vi "DSF.Engine.Builder.Buffer.Parse.vi"(6 "VS Channel Buffer in":dbl[](array[numeric]), 7 "Data Type Buffers in":T5, 8 "error in (no error)":errorcluster, 10 "command":T3, 11 "Builder in":refnum<class "DSF.Engine.Builder.lvclass">) -> (0 "error out":errorcluster, 2 "response":T1, 3 "Builder out":refnum<class "DSF.Engine.Builder.lvclass">, 4 "VS Channel Buffer out":dbl[](array[numeric]), 5 "Data Type Buffers out":T5)   [LabVIEW 2016, in "DSF.Engine.lvlib" / "DSF.Engine.Builder.lvclass"]
uses:
  DSF.Engine.Builder.lvclass
  Typedefs/DSF.Engine.Typedefs.Type Buffers.ctl
  Interface/DSF.Engine.Interface.Builder.Command Data.ctl
  Interface/DSF.Engine.Interface.Builder.Command.ctl
  Interface/DSF.Engine.Interface.Builder.Response Data.ctl
  Interface/DSF.Engine.Interface.Builder.Response.ctl
  DSF.Engine.Builder.lvclass/DSF.Engine.Builder.ctl
  Cache/DSF.Engine.Memory.Cache.Plugin.lvclass/DSF.Engine.Memory.Cache.Plugin.ctl
  Cache/DSF.Engine.Memory.Cache.Transfer Group.lvclass/DSF.Engine.Memory.Cache.Transfer Group.ctl
  Cache/DSF.Engine.Memory.Cache.Transfer.lvclass/DSF.Engine.Memory.Cache.Transfer.ctl
  Shared/Classes/Transfer/DSF.Shared.Configuration.Transfer.lvclass/DSF.Shared.Configuration.Transfer.ctl
  Cache/DSF.Engine.Memory.Cache.Transfer Group.Get Transfer Caches.vi
  Cache/DSF.Engine.Memory.Cache.Plugin.Get Transfer Group Caches.vi
  Buffer/DSF.Engine.Memory.Buffer.lvclass
  Pointer/DSF.Engine.Pointer.VS Channels.lvclass
  Cache/DSF.Engine.Memory.Cache.Transfer Group.lvclass
  Cache/DSF.Engine.Memory.Cache.Framework.lvclass
  Cache/DSF.Engine.Memory.Cache.Plugin.lvclass
  Cache/DSF.Engine.Memory.Cache.Transfer.lvclass
  Shared/Classes/Transfer/DSF.Shared.Configuration.Transfer.lvclass
  Interface/DSF.Engine.Interface.Builder.lvclass
  DSF.Engine.lvlib
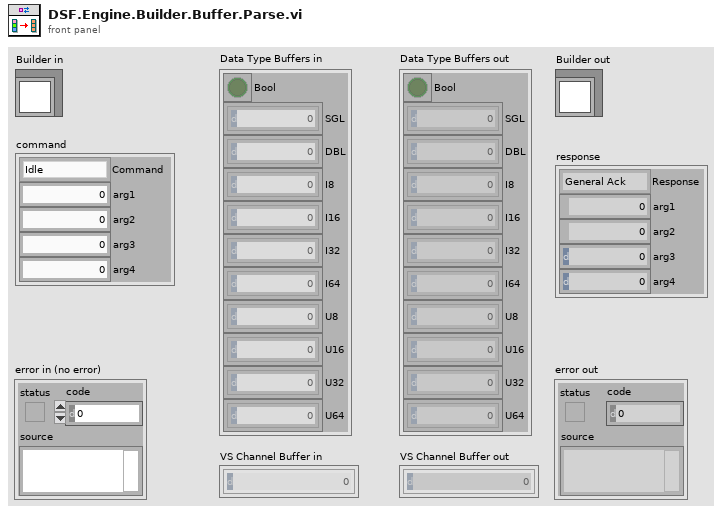
[diagram p1: front panel]
types:
  T1 = typedef "DSF.Engine.lvlib/DSF.Engine.Interface.Builder.lvclass/DSF.Engine.Interface.Builder.Response Data.ctl" = cluster{"Response":T2, "arg1":i32, "arg2":i32, "arg3":i32, "arg4":i32}
  T2 = typedef "DSF.Engine.lvlib/DSF.Engine.Interface.Builder.lvclass/DSF.Engine.Interface.Builder.Response.ctl" = enum8{"General Ack", "Initialize Complete", "Build Complete", "Parse Complete", "Shutdown Ack"}
  T3 = typedef "DSF.Engine.lvlib/DSF.Engine.Interface.Builder.lvclass/DSF.Engine.Interface.Builder.Command Data.ctl" = cluster{"Command":T4, "arg1":i32, "arg2":i32, "arg3":i32, "arg4":i32}
  T4 = typedef "DSF.Engine.lvlib/DSF.Engine.Interface.Builder.lvclass/DSF.Engine.Interface.Builder.Command.ctl" = enum8{"Idle", "Initialize", "Build Buffer", "Parse Buffer", "Shutdown"}
  T5 = typedef "DSF.Engine.lvlib/DSF.Engine.Typedefs.Type Buffers.ctl" = cluster{"Bool":bool[], "SGL":sgl[], "DBL":dbl[], "I8":i8[], "I16":i16[], "I32":i32[], "I64":i64[], "U8":u8[], "U16":u16[], "U32":u32[], "U64":u64[]}
  T6 = typedef "DSF.Engine.lvlib/DSF.Engine.Builder.lvclass/DSF.Engine.Builder.Command.Build-Parse.ctl" = cluster{"unused":u8, "Plugin ID":i32, "Transfer Group ID":i32, "Transfer ID":i32, "unused":i32}
  T7 = typedef "DSF.Shared.lvlib/DSF.Shared.Typedefs.Configuration.Transfer.Channel Block Descriptor.ctl" = cluster{"First Channel Descriptor":T8, "count":u64, "vs channel index":u64}
  T8 = typedef "DSF.Shared.lvlib/DSF.Shared.Typedefs.Configuration.Transfer.Channel Descriptor.ctl" = cluster{"Channel Parameters":T9, "VS Channel Ref":T11}
  T9 = typedef "DSF.Shared.lvlib/DSF.Shared.Typedefs.Configuration.Transfer.Channel Parameters.ctl" = cluster{"offset":u64, "data type":T10}
  T10 = typedef "DSF.Shared.lvlib/DSF.Shared.Typedefs.Data Type.ctl" = enum8{"Bool", "SGL", "DBL", "I8", "I16", "I32", "I64", "U8", "U16", "U32", "U64"}
  T11 = typedef "Custom Device API.lvlib/Custom Device Item Ref.ctl" = u64
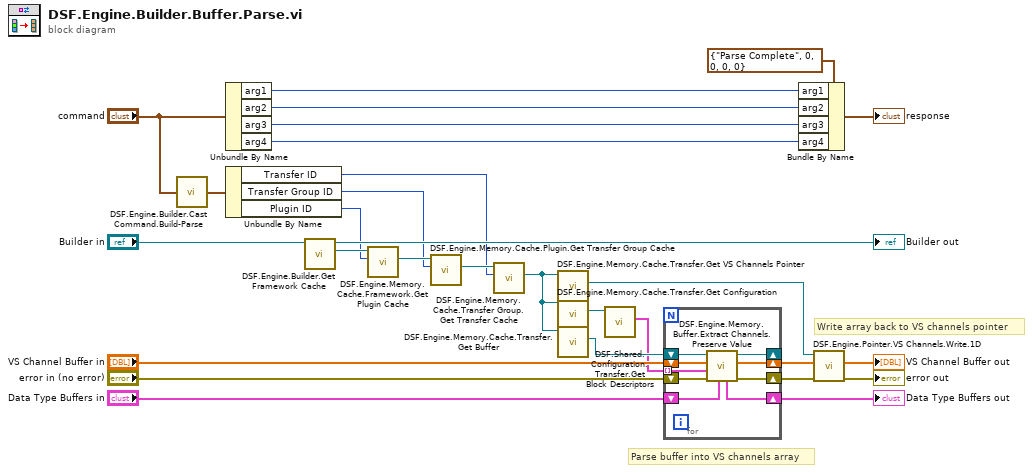
[diagram p0: block diagram]
diagram:
  # "Parse buffer into VS channels array"
  # "Write array back to VS channels pointer"
  n1 = call "DSF.Engine.Builder.Cast Command.Build-Parse.vi"("command"="command") -> ("build/parse command"=w8:T6)
  n2 = Unbundle By Name("command") -> ("arg1"=w5:i32, "arg2"=w6:i32, "arg3"=w2:i32, "arg4"=w1:i32)
  n3 = Unbundle By Name(w8) -> ("Transfer ID"=w19:i32, "Transfer Group ID"=w18:i32, "Plugin ID"=w20:i32)
  n4 = call "DSF.Engine.Builder.Get Framework Cache.vi"("Builder in"="Builder in") -> ("Framework Cache"=w24:refnum<class "DSF.Engine.Memory.Cache.Framework.lvclass">, "Builder out"=→"Builder out":refnum<class "DSF.Engine.Builder.lvclass">)  [unwired: 9 in]
  n5 = call "DSF.Engine.Memory.Cache.Framework.Get Plugin Cache.vi"("Plugin ID"=w20, "Framework Cache in"=w24) -> ("Plugin Cache"=w23:refnum<class "DSF.Engine.Memory.Cache.Plugin.lvclass">)  [unwired: 8 in, 1 out]
  n6 = call "DSF.Engine.Memory.Cache.Plugin.Get Transfer Group Cache.vi"("Transfer Group ID"=w18, "Plugin Cache in"=w23) -> ("Transfer Group Cache"=w22:refnum<class "DSF.Engine.Memory.Cache.Transfer Group.lvclass">)  [unwired: 8 in, 1 out]
  n7 = call "DSF.Engine.Memory.Cache.Transfer Group.Get Transfer Cache.vi"("Transfer ID"=w19, "Transfer Group Cache in"=w22) -> ("Transfer Cache"=w12:refnum<class "DSF.Engine.Memory.Cache.Transfer.lvclass">)  [unwired: 8 in, 1 out]
  n8 = call "DSF.Engine.Memory.Cache.Transfer.Get VS Channels Pointer.vi"("Transfer Cache in"=w12) -> ("VS Channels Pointer"=w11:refnum<class "DSF.Engine.Pointer.VS Channels.lvclass">)  [unwired: 9 in, 1 out]
  n9 = call "DSF.Engine.Memory.Cache.Transfer.Get Configuration.vi"("Transfer Cache in"=w12) -> ("Transfer Configuration"=w21:refnum<class "DSF.Shared.Configuration.Transfer.lvclass">)  [unwired: 9 in, 1 out]
  n10 = call "DSF.Engine.Memory.Cache.Transfer.Get Buffer.vi"("Transfer Cache in"=w12) -> ("Buffer"=w10:refnum<class "DSF.Engine.Memory.Buffer.lvclass">)  [unwired: 9 in, 1 out]
  n11 = call "DSF.Shared.Configuration.Transfer.Get Block Descriptors.vi"("Transfer Configuration in"=w21) -> ("Channel Blocks"=w9:T7[])  [unwired: 8 in, 2 out]
  n12 = for {
    shift-right: [w36] -> w28
    shift-left: "VS Channel Buffer in" -> [w37]
    shift-right: [w35] -> w25
    shift-left: "error in (no error)" -> [w38]
    shift-right: [w32] -> w26
    shift-left: "Data Type Buffers in" -> [w33]
    shift-right: [w31] -> _
    shift-left: w10 -> [w34]
    tunnel: w9 -> [w30] mode=indexing
    n13 = call "DSF.Engine.Memory.Buffer.Extract Channels.Preserve Value.vi"("Data Type Buffers in"=w33, "error in (no error)"=w38, "Channel Block"=w30, "VS Channels Array in"=w37, "Buffer in"=w34) -> ("error out"=w35:errorcluster, "VS Channels Array out"=w36:dbl[], "Buffer out"=w31:refnum<class "DSF.Engine.Memory.Buffer.lvclass">, "Data Type Buffers out"=w32:T5)  [unwired: 3 in]
  }
  "Data Type Buffers out" <- w26
  n14 = Bundle By Name(cluster=T1 {"Response"=enum."Parse Complete", "arg1"=0, "arg2"=0, "arg3"=0, "arg4"=0} ("response"), "arg1"=w5, "arg2"=w6, "arg3"=w2, "arg4"=w1) -> (→"response":T1)
  n15 = call "DSF.Engine.Pointer.VS Channels.Write.1D.vi"("error in (no error)"=w25, "Channels Array in"=w28, "VS Channels Pointer in"=w11) -> ("error out"=→"error out":errorcluster, "Channels Array out"=→"VS Channel Buffer out":dbl[])  [unwired: 5 in, 2 out]
